vi "XML_EEG_waveformToHexString.vi"(8 "error in (no error)":errorcluster, 11 "Analog waveform in":waveform(dbl)) -> (0 "error out":errorcluster, 3 "HexString out":string)   [LabVIEW 2016, in "XML_EEG_File_Parser.lvlib"]
uses:
  XML_EEG_File_Parser.lvlib
panel:
  # "This VI is a part of BCI Design library, http://www.ru-bci.org \nCopyright © 2020, Sotnikov Peter, All rights reserved. License: GNU GPLv3"
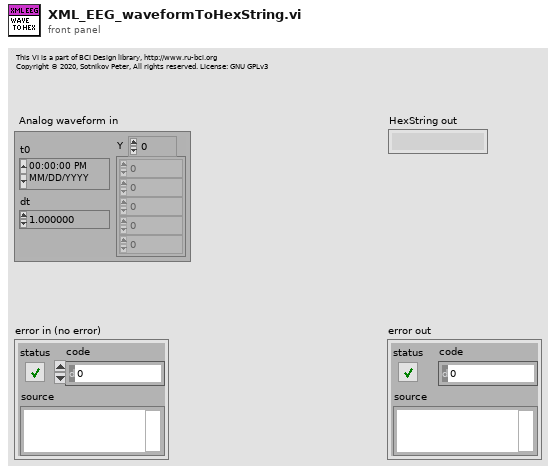
[diagram p1: front panel]
types:
  T1 = enum16{"big-endian, network order", "native, host order", "little-endian"}
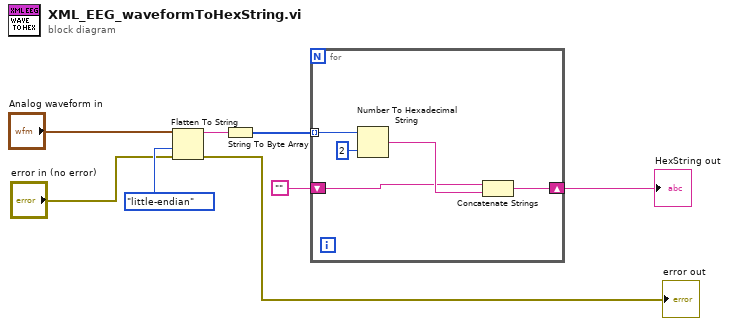
[diagram p0: block diagram]
diagram:
  n1 = Flatten To String(anything="Analog waveform in", byte order (0:big-endian, network order)=T1."little-endian", error in (no error)="error in (no error)") -> (data string=w5:string, error out=→"error out":errorcluster)  [unwired: 1 in, 1 out]
  n2 = String To Byte Array(string=w5) -> (unsigned byte array=w4:u8[])
  n3 = for {
    tunnel: w4 -> [w13] mode=indexing
    shift-right: [w11] -> w2
    shift-left: "" -> [w10]
    n4 = Number To Hexadecimal String(1:i16 2 ("width (-)"), 2:w13) -> (0:w12:string)
    n5 = Concatenate Strings(w10, w12) -> (w11:string)
  }
  "HexString out" <- w2
